vi "setServoDefaultPosition.vi"() -> ()   [LabVIEW 2011]
uses:
  stopServos.vi
panel:
  in  "done setting position":bool
  in  "channel":u8
  in  "servo custom position":u16(knob)=750 min=260 max=1150 step=1 scale=260.0..1150.0
  out "error out":errorcluster
  out "serial status":u32(colorbox)
  in  "VISA resource name":refnum<visa-resource-name>="COM3"
  in  "task":u16(ring) items=["Set custom position", "Enable custom position", "Disable custom position"]
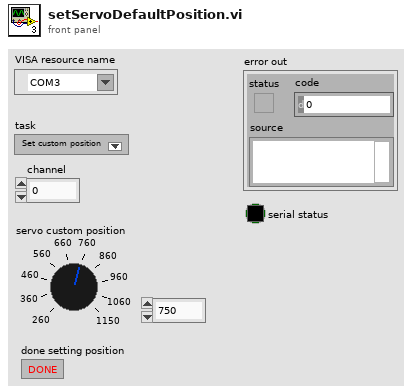
[diagram p1: front panel]
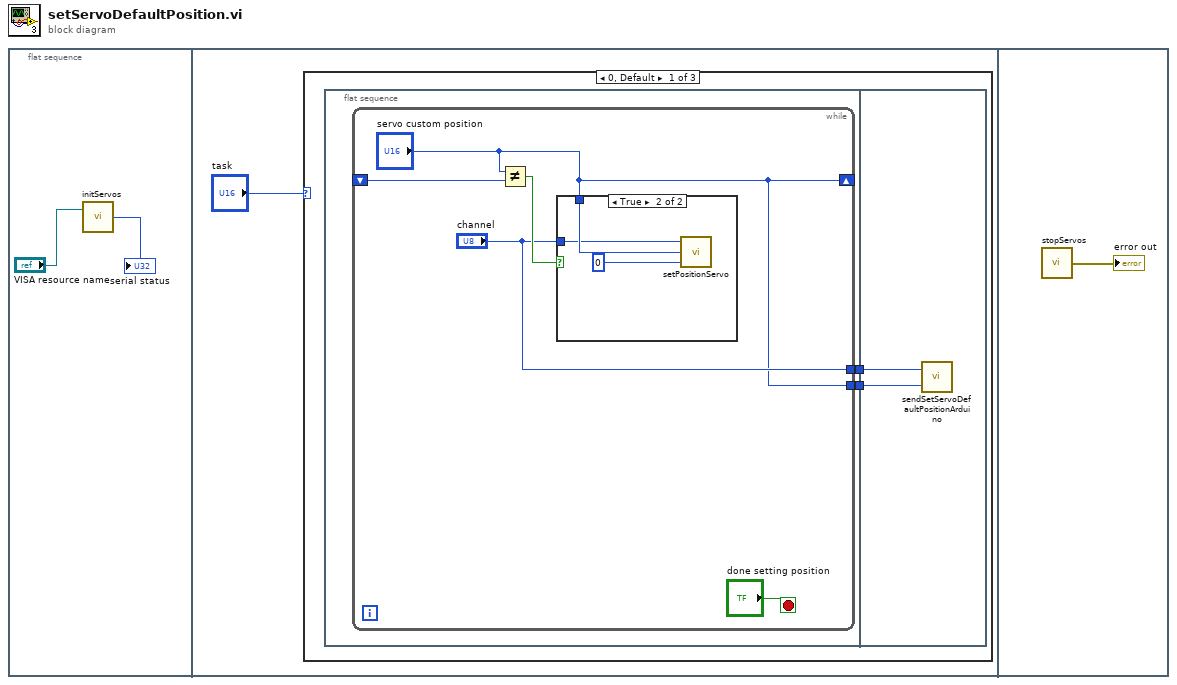
[diagram p0: block diagram]
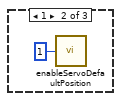
[diagram p3: hidden frame]
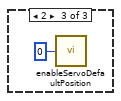
[diagram p4: hidden frame]
diagram:
  n1 = flat-sequence {
    frame #0 {
      n2 = call "initServos.vi"("VISA resource name"="VISA resource name") -> ("serial status"=→"serial status":u32)  [unwired: 1 in]
    }
    frame #1 {
      n3 = case shown="0, Default" "task" {
        frame 0, Default {
          n4 = flat-sequence {
            tunnel: [w7] -> w5
            tunnel: [w6] -> w4
            tunnel: w5 -> [w17]
            tunnel: w4 -> [w16]
            frame #0 {
              n5 = while {
                shift-right: ["servo custom position"] -> _
                shift-left: _ -> [w12]
                tunnel: ["channel"] -> w7
                tunnel: ["servo custom position"] -> w6
                stop <- "done setting position" stop-if-true
                n6 = Not Equal?(x="servo custom position", y=w12) -> (x != y?=w11:bool)
                n7 = case shown="True" w11 {
                  tunnel: "servo custom position" -> [_ w14]
                  tunnel: "channel" -> [_ w13]
                  frame False {
                  }
                  frame True {
                    n8 = call "setPositionServo.vi"("speed"=u8 0, "servo position"=w14, "channel"=w13) -> ()
                  }
                }
              }
            }
            frame #1 {
              n9 = call "sendSetServoDefaultPositionArduino.vi"("servo position"=w16, "channel"=w17) -> ()  [unwired: 1 in]
            }
          }
        }
        frame 1 {
          n10 = call "enableServoDefaultPosition.vi"("enable bit"=u8 1) -> ()  [unwired: 1 in]
        }
        frame 2 {
          n11 = call "enableServoDefaultPosition.vi"("enable bit"=u8 0) -> ()  [unwired: 1 in]
        }
      }
    }
    frame #2 {
      n12 = call "stopServos"() -> ("error out"=→"error out":errorcluster)  [unwired: 2 in]
    }
  }
